vi "testFlattenAngularVelocityToXML.vi"() -> ()   [LabVIEW 2012, in "UnitsAndXML.lvlib"]
uses:
  <userlib>/Common/UnitsAndXML/UnitsAndXML.lvlib
  <userlib>/Common/UnitsAndXML/FlattenItemWithUnitToXML/FlattenAngularVelocityToXML/AngularVelocityUnit.ctl
  <userlib>/Common/UnitsAndXML/FlattenItemWithUnitToXML/FlattenAngularVelocityToXML/typeMethods/flattenAngularVelocityToXML_Array.vi
  <userlib>/Common/UnitsAndXML/FlattenItemWithUnitToXML/FlattenAngularVelocityToXML/typeMethods/flattenAngularVelocityToXML_Scalar.vi
panel:
  out "error out":errorcluster
  in  "angularVelocityUnitInXML":T1
  out "xmlStringArray":string
  out "xmlStringScalar":string
  in  "angularVelocity":dbl[unit][](array[numeric])=[0.2617993877991494, 0.5235987755982988, 0.7853981633974483, 1.0471975511965976]
  in  "angularVelocity":dbl[unit]=0.2617993877991494
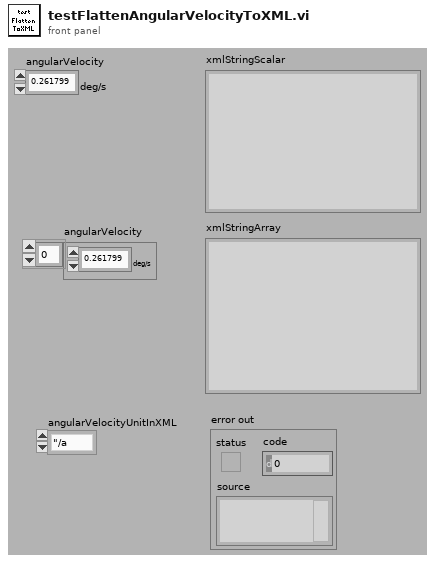
[diagram p1: front panel]
types:
  T1 = typedef "UnitsAndXML.lvlib/AngularVelocityUnit.ctl" = enum16{"\"/a", "deg/s", "\"/s"}
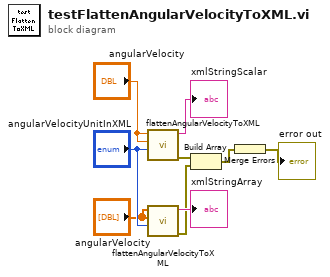
[diagram p0: block diagram]
diagram:
  n1 = call-poly <userlib>:"flattenAngularVelocityToXML.vi"("angularVelocityUnitInXML"="angularVelocityUnitInXML", "anuglarVelocityAgain"="angularVelocity", "angularVelocity"="angularVelocity") -> ("error out"=w6:errorcluster, "xmlString"=→"xmlStringScalar":string)  [unwired: 7 in]
  n2 = call-poly <userlib>:"flattenAngularVelocityToXML.vi"("angularVelocityUnitInXML"="angularVelocityUnitInXML", "angularVelocityAgain"="angularVelocity", "angularVelocity"="angularVelocity") -> ("error out"=w1:errorcluster, "xmlString"=→"xmlStringArray":string)  [unwired: 7 in]
  n3 = Build Array(w6, w1) -> (w7:errorcluster[])
  n4 = Merge Errors(w7) -> (→"error out":errorcluster)
